vi "GetAxisErrors.vi"(4 "error in (no error)":errorcluster, 7 "axis in":cluster{"keyHandle":u32, "nodeId":u16}={"keyHandle"=0, "nodeId"=1}) -> (0 "error out":errorcluster, 2 "axis errors":u32[](array[numeric]) format="%x", 3 "axis out":cluster{"keyHandle":u32, "nodeId":u16}={"keyHandle"=0, "nodeId"=1})   [LabVIEW 2018]
doc: "<B>GetAxisErrors</B> reads the number of error and returns the error code(-s) in an array."
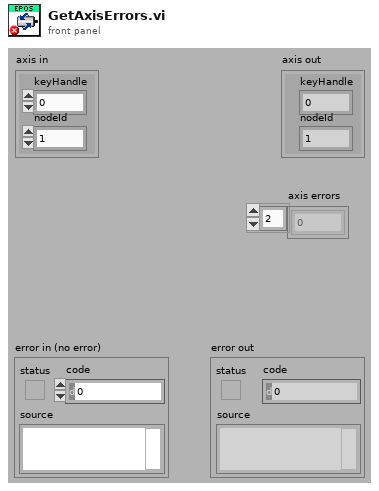
[diagram p1: front panel]
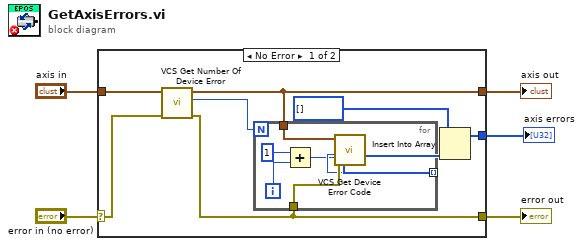
[diagram p0: block diagram]
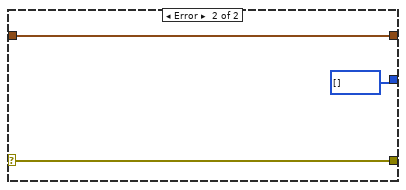
[diagram p2: hidden frame]
diagram:
  n1 = case shown="No Error" "error in (no error)" {
    selector: "error in (no error)" -> [w12 w22]
    tunnel: [w11 w22] -> w4
    tunnel: [w10 w21] -> w3
    tunnel: "axis in" -> [w13 w21]
    tunnel: [w8 u32[] []] -> w1
    frame No Error {
      n2 = call "VCS Get Number Of Device Error.vi"("error in (no error)"=w12, "axis in"=w13) -> ("error out"=w11:errorcluster, "NbDeviceError"=w9:u8, "axis out"=w10:cluster{"keyHandle":u32, "nodeId":u16})  [unwired: 7 in]
      n3 = for {
        N: w9 -> [_]
        tunnel: w11 -> [w19]
        tunnel: w10 -> [w18]
        tunnel: [w17] -> w7 mode=indexing
        i -> [w16]
        n4 = Add(x=1, y=w16) -> (x+y=w15:i32)
        n5 = call "VCS Get Device Error Code.vi"("error in (no error)"=w19, "Error Number"=w15, "axis In"=w18) -> ("Error Code"=w17:u32)  [unwired: 6 in, 2 out]
      }
      n6 = Insert Into Array(array=u32[] [], new element=w7) -> (w8:u32[])  [unwired: 1 in]
    }
    frame Error {
    }
  }
  "error out" <- w4
  "axis out" <- w3
  "axis errors" <- w1
